vi "Degrees to Microsteps (SubVI).vi"(4 "Degrees":dbl) -> (1 "Microsteps":dbl)   [LabVIEW 2012]
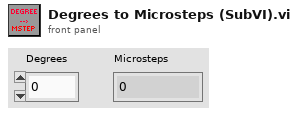
[diagram p1: front panel]
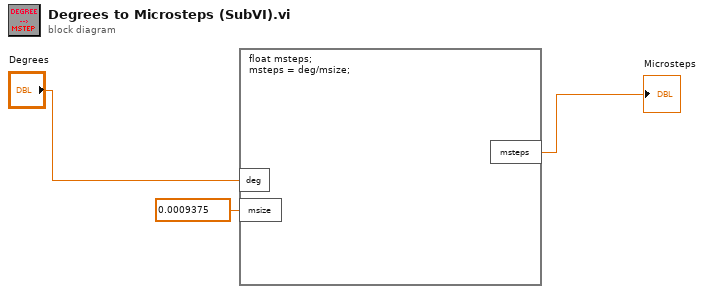
[diagram p0: block diagram]
diagram:
  n1 = formula code="float msteps;\nmsteps = deg/msize;"("deg"="Degrees", "msize"=0.0009375 ("input variable")) -> ("msteps"=→"Microsteps":dbl)
